vi "Initialize.vi"(8 "error in (no error)":errorcluster, 9 "Host IP Address":string, 10 "Scanner IP Address":string, 11 "PF_API in":refnum<class "PF_API.lvclass">) -> (0 "error out":errorcluster, 3 "PF_API out":refnum<class "PF_API.lvclass">)   [LabVIEW 2019, in "PF_API.lvclass"]
doc: "Initializes the communication with the Scanner."
uses:
  PF_API.lvclass
  PF_API.lvclass/PF_API.ctl
  <vilib>/httpClient/LabVIEWHTTPClient.lvlib
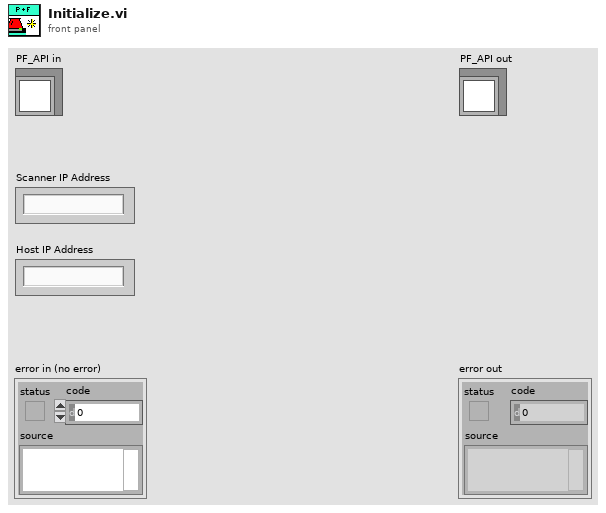
[diagram p1: front panel]
types:
  T1 = cluster{"version_major":i32, "version_minor":i32}
  T2 = typedef "LabVIEWHTTPClient.lvlib/ClientHandle.ctl" = refnum<k1>
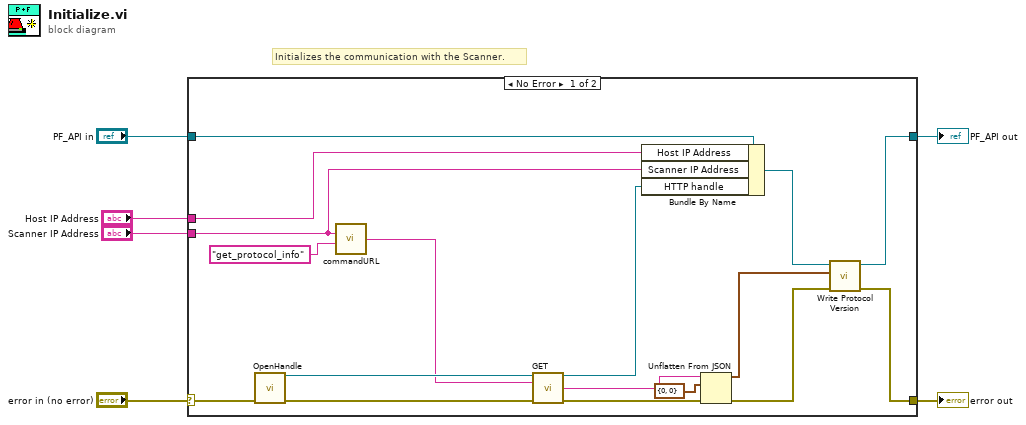
[diagram p0: block diagram]
diagram:
  # "Initializes the communication with the Scanner."
  n1 = case shown="No Error" "error in (no error)" {
    selector: "error in (no error)" -> [w21 w25]
    tunnel: [w11 w25] -> w5
    tunnel: [w13 w24] -> w3
    tunnel: "PF_API in" -> [w23 w24]
    tunnel: "Scanner IP Address" -> [w14 _]
    tunnel: "Host IP Address" -> [w15 _]
    frame No Error {
      n2 = call <vilib>:"OpenHandle.vi"("error in (no error)"=w21) -> ("client handle out"=w19:T2, "error out"=w20:errorcluster)  [unwired: 13 in]
      n3 = call "commandURL.vi"("Command String"="get_protocol_info", "Scanner IP Address"=w14) -> ("Command URL"=w18:string)  [unwired: 4 in]
      n4 = call <vilib>:"GET.vi"("client handle"=w19, "url"=w18, "error in (no error)"=w20) -> ("client handle out"=w16:T2, "body"=w9:string, "error out"=w12:errorcluster)  [unwired: 9 in, 1 out]
      n5 = Bundle By Name(cluster=w23, "Host IP Address"=w15, "Scanner IP Address"=w14, "HTTP handle"=w16) -> (w17:refnum<class "PF_API.lvclass">)
      n6 = Unflatten From JSON(JSON string=w9, type and defaults=T1 {"version_major"=0, "version_minor"=0} ("Protocol Version"), error in (no error)=w12) -> (value=w7:T1, error out=w10:errorcluster)  [unwired: 4 in]
      n7 = call "Write Protocol Version.vi"("error in (no error)"=w10, "Protocol Version"=w7, "PF_API in"=w17) -> ("error out"=w11:errorcluster, "PF_API out"=w13:refnum<class "PF_API.lvclass">)  [unwired: 7 in]
    }
    frame Error {
    }
  }
  "error out" <- w5
  "PF_API out" <- w3
